vi "Select Single Variable.vi"(8 "error in (no error)":errorcluster, 10 "varName":string, 11 "muExpr in":refnum<class "muExpr.lvclass">) -> (0 "error out":errorcluster, 3 "muExpr out":refnum<class "muExpr.lvclass">)   [LabVIEW 2015, in "muParser.lvlib" / "muExpr.lvclass"]
uses:
  muExpr.lvclass
  muExpr.lvclass/muExpr.ctl
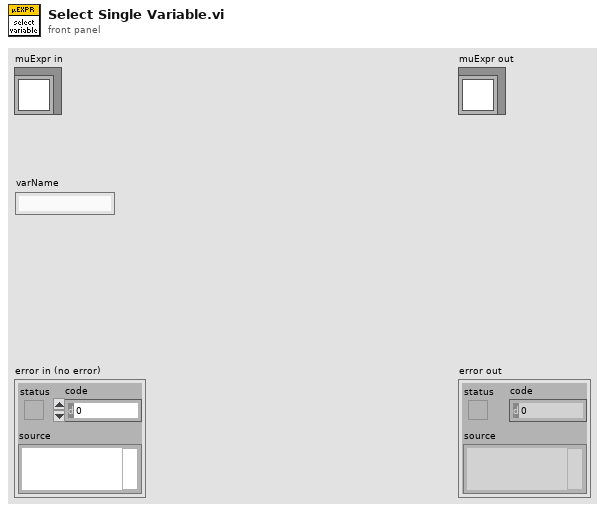
[diagram p1: front panel]
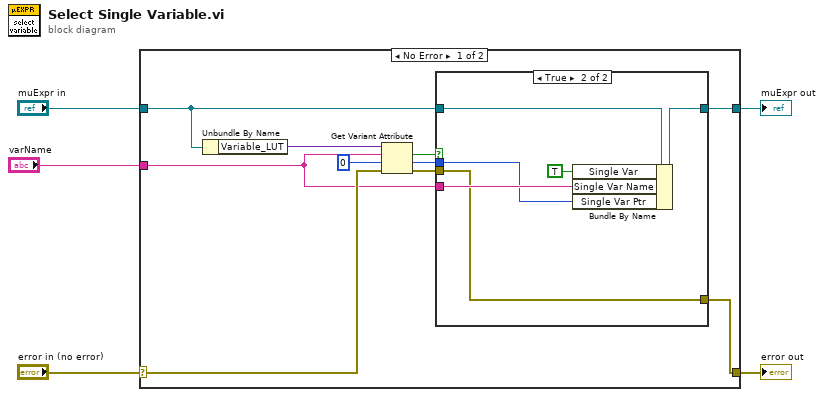
[diagram p0: block diagram]
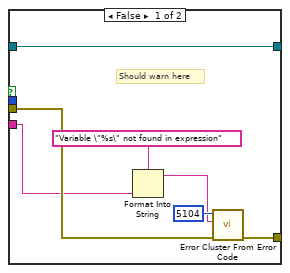
[diagram p2: hidden frame]
diagram:
  n1 = case shown="No Error" "error in (no error)" {
    selector: "error in (no error)" -> [w11 w30]
    tunnel: [w6 w30] -> w4
    tunnel: [w8 w29] -> w2
    tunnel: "muExpr in" -> [w10 w29]
    tunnel: "varName" -> [w9 _]
    frame No Error {
      n2 = Unbundle By Name(w10) -> ("Variable_LUT"=w15:variant)
      n3 = Get Variant Attribute(Variant=w15, name=w9, default value (empty Variant)=u64 0, error in=w11) -> (found=w14:bool, value=w12:u64, error out=w7:errorcluster)  [unwired: 1 out]
      n4 = case shown="True" w14 {
        tunnel: w12 -> [_ w25]
        tunnel: w10 -> [w22 w28]
        tunnel: w9 -> [w18 w26]
        tunnel: [w22 w24] -> w8
        tunnel: w7 -> [w21 w23]
        tunnel: [w16 w23] -> w6
        frame False {
          # "Should warn here"
          n5 = Format Into String(format string="Variable \"%s\" not found in expression" ("error message (\"\")"), w18) -> (resulting string=w17:string)  [unwired: 2 in, 1 out]
          n6 = call <vilib>:"Error Cluster From Error Code.vi"("error in (no error)"=w21, "error message (\"\")"=w17, "error code (0)"=5104) -> ("error out"=w16:errorcluster)  [unwired: 6 in]
        }
        frame True {
          n7 = Bundle By Name(cluster=w28, "Single Var"=TRUE, "Single Var Name"=w26, "Single Var Ptr"=w25) -> (w24:refnum<class "muExpr.lvclass">)
        }
      }
    }
    frame Error {
    }
  }
  "error out" <- w4
  "muExpr out" <- w2
